vi "String_StripNullValues.vi"(11 "str in":string) -> (3 "str (stripped)":string)   [LabVIEW 2022 SP3, in "hse-misc.lvlib"]
doc: "Removes all NULL values from a string\n\n\n\n____\nHAMPEL SOFTWARE ENGINEERING v3.8.0 (2023-12-18 14:41)"
uses:
  hse-misc.lvlib
  <vilib>/Utility/error.llb/Trim Whitespace One-Sided.vi
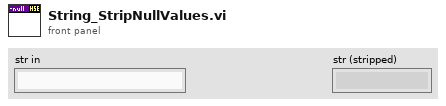
[diagram p1: front panel]
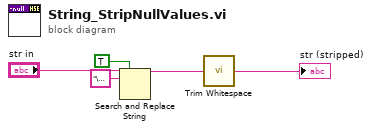
[diagram p0: block diagram]
diagram:
  n1 = Search and Replace String(replace all?=TRUE ("replace all? (F)"), input string="str in", search string="\u0000") -> (result string=w2:string)  [unwired: 5 in, 3 out]
  n2 = call <vilib>:"Trim Whitespace.vi"("string"=w2) -> ("trimmed string"=→"str (stripped)":string)  [unwired: 1 in]
